vi "USB_Communication.vi"(8 "error in (no error)":errorcluster, 9 "number":i32, 10 "string":string, 11 "APS PORT":refnum<visa-resource-name>) -> (0 "error out":errorcluster, 2 "read buffer":string, 3 "APS PORT Out":refnum<visa-resource-name>)   [LabVIEW 2025]
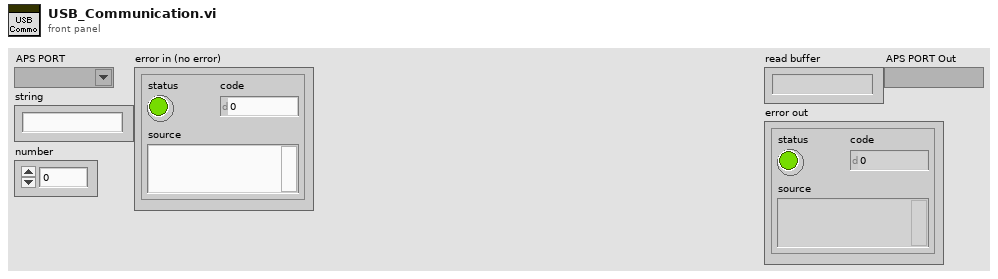
[diagram p1: front panel]
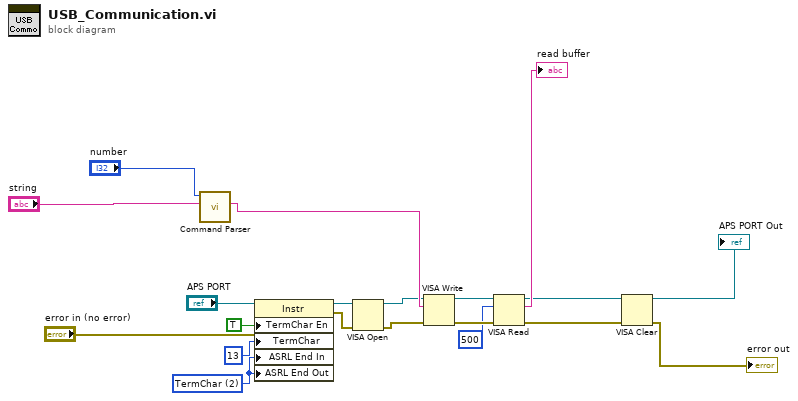
[diagram p0: block diagram]
diagram:
  w15 = u16 2 items=["None", "Last Bit", "TermChar", "Break"] ("Serial Settings:End Mode for Writes")
  n1 = call "Command Parser.vi"("Task IN"="string", "Numeric"="number") -> ("Task Out"=w12:string)  [unwired: 9 in]
  n2 = property class="Instr"(reference="APS PORT", error in="error in (no error)", "TermChar En"=TRUE ("Message Based Settings:Termination Character Enable"), "TermChar"=u8 13 ("Message Based Settings:Termination Character"), "ASRL End In"=w15, "ASRL End Out"=w15) -> (reference out=w20:refnum<visa-resource-name>, error out=w19:errorcluster)
  n3 = VISA Open(error in (no error)=w19, VISA resource name=w20) -> (VISA resource name=w11:refnum<visa-resource-name>, error out=w10:errorcluster)  [unwired: 3 in]
  n4 = VISA Write(VISA resource name=w11, write buffer=w12, error in (no error)=w10) -> (VISA resource name out=w8:refnum<visa-resource-name>, error out=w9:errorcluster)  [unwired: 1 out]
  n5 = VISA Read(VISA resource name=w8, byte count=u32 500, error in (no error)=w9) -> (VISA resource name out=w6:refnum<visa-resource-name>, read buffer=→"read buffer":string, error out=w5:errorcluster)  [unwired: 1 out]
  n6 = VISA Clear(VISA resource name=w6, error in (no error)=w5) -> (VISA resource name out=→"APS PORT Out":refnum<visa-resource-name>, error out=→"error out":errorcluster)
